vi "Do ReferenceMove.vi"(8 "error in (no error)":errorcluster, 10 "AxisNumber":u8, 11 "CS++IEFWerner in":refnum<class "CS++IEFWerner.lvclass">) -> (0 "error out":errorcluster, 3 "CS++IEFWerner out":refnum<class "CS++IEFWerner.lvclass">)   [LabVIEW 2015, in "CS++IEFWerner.lvlib" / "CS++IEFWerner.lvclass"]
doc: "Starts a movement to the reference switch of this axis. Once the motor reaches the reference switch it should slowly move down from the switch and stop. Afterwards the internal step counter is set to zero. \n\nThe main purpose of this function is to calibrate the motor.\n\nA reference Move of the IEFWerner is different: It has to be started from a different thread in order not to stop the complete actor from working."
uses:
  CS++IEFWerner.lvclass
  CS++IEFWerner.lvclass/CS++IEFWerner.ctl
  instr.lib/IEF-pac/IEF Werner.lvlib
  CSPP_DeviceBase/CS++Motor/CS++Motor.lvclass
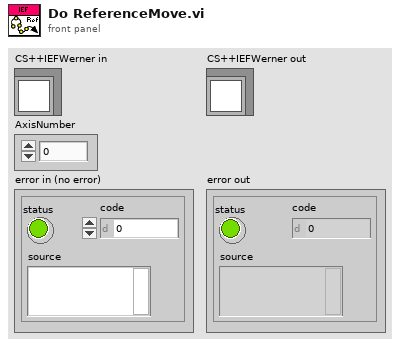
[diagram p1: front panel]
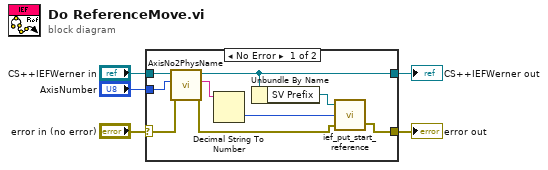
[diagram p0: block diagram]
diagram:
  n1 = case shown="No Error" "error in (no error)" {
    selector: "error in (no error)" -> [w9 w15]
    tunnel: "CS++IEFWerner in" -> [w11 w16]
    tunnel: [w13 w15] -> w2
    tunnel: [w6 w16] -> w4
    tunnel: "AxisNumber" -> [w7 _]
    frame No Error {
      n2 = call "AxisNo2PhysName.vi"("error in (no error)"=w9, "AxisNumber"=w7, "CS++Motor in"=w11) -> ("error out"=w8:errorcluster, "PhysicalChannelName"=w12:string, "CS++Motor out"=w6:refnum<class "CS++IEFWerner.lvclass">)  [unwired: 6 in]
      n3 = Decimal String To Number(string=w12) -> (number=w10:i32)  [unwired: 2 in, 1 out]
      n4 = Unbundle By Name(w6) -> ("SV Prefix"=w14:refnum<k21>)
      n5 = call "ief_put_start_reference.vi"("error in (no error)"=w8, "Axis Number"=w10, "Tagprefix in"=w14) -> ("error out (no error)"=w13:errorcluster)  [unwired: 1 out]
    }
    frame Error {
    }
  }
  "error out" <- w2
  "CS++IEFWerner out" <- w4
